vi "计数I2C config.vi"(1 "VISA":refnum<visa-resource-name>="COM6") -> (0 "VISA资源名称输出":refnum<visa-resource-name>)   [LabVIEW 2011]
uses:
  <vilib>/Instr/_visa.llb/VISA Configure Serial Port (Instr).vi
panel:
  in  "Error in":errorcluster
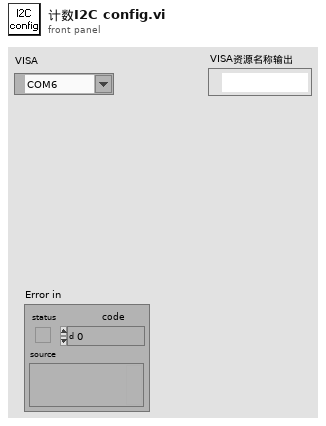
[diagram p1: front panel]
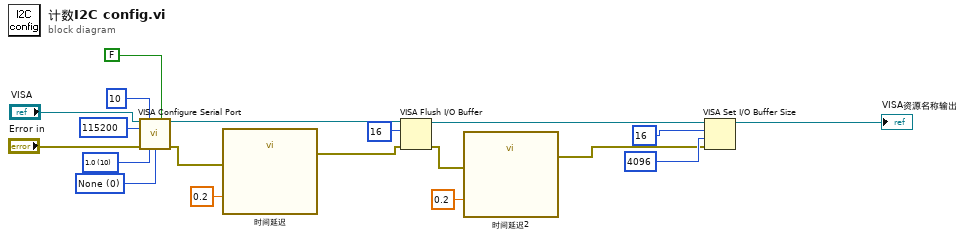
[diagram p0: block diagram]
diagram:
  w11 = u16 0 items=["None", "XON/XOFF", "RTS/CTS", "XON/XOFF & RTS/CTS", "DTR/DSR", "XON/XOFF & DTR/DSR"] ("flow control (0:none)")
  w16 = u16 10 items=["1.0"=10, "1.5"=15, "2.0"=20] ("stop bits (10: 1 bit)")
  n1 = call-poly "VISA Configure Serial Port"("VISA resource name"="VISA", "timeout (10sec)"=u32 10 ("timeout"), "Enable Termination\nChar (T)"=FALSE ("Enable Termination\nChar (T)"), "baud rate (9600)"=u32 115200 ("baud rate"), "error in (no error)"="Error in", "stop bits (10: 1 bit)"=w16, "flow control (0:none)"=w11) -> ("VISA resource name out"=w10:refnum<visa-resource-name>, "error out"=w7:errorcluster)  [unwired: 7 in]
  n2 = call "时间延迟"("error in (no error)"=w7, "Delay Time (s)"=0.2) -> ("error out"=w6:errorcluster)  [unwired: 9 in]
  n3 = VISA Flush I/O Buffer(VISA resource name=w10, mask (16)=u16 16, error in (no error)=w6) -> (VISA resource name out=w14:refnum<visa-resource-name>, error out=w4:errorcluster)
  n4 = call "时间延迟2"("error in (no error)"=w4, "Delay Time (s)"=0.2) -> ("error out"=w3:errorcluster)  [unwired: 9 in]
  n5 = VISA Set I/O Buffer Size(VISA resource name=w14, mask (16)=u16 16, size (4096)=u32 4096 ("size (0)"), error in (no error)=w3) -> (VISA resource name out=→"VISA资源名称输出":refnum<visa-resource-name>)  [unwired: 1 out]
